vi "Move Addon Settings.vi"(8 "error in (no error)":errorcluster, 11 "Section Ref in":T1 format="%.0x") -> (0 "error out":errorcluster, 3 "Parent Ref out":T1 format="%.0x")   [LabVIEW 2023, in "J1939 Addon System Explorer.lvlib"]
uses:
  J1939 Addon System Explorer.lvlib
  <vilib>/NI VeriStand/Custom Device API/Custom Device Item Ref.ctl
  Addon Shared/SubVIs/Constants.vi
  <vilib>/NI VeriStand/Custom Device API/Custom Device API.lvlib
  Addon Shared/J1939 Addon Shared.lvlib
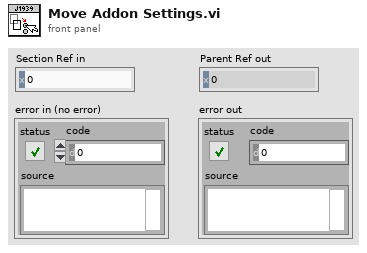
[diagram p1: front panel]
types:
  T1 = typedef "Custom Device API.lvlib/Custom Device Item Ref.ctl" = u64
  T2 = typedef "J1939 Addon Shared.lvlib/SPN Properties.ctl" = cluster{"Bytes":u32, "ScaleFac":dbl, "ScaleOff":dbl}
  T3 = cluster{"Name":string, "ID":u32, "Signal List":cluster{"Name":string, "SPN":T2}[]}[]
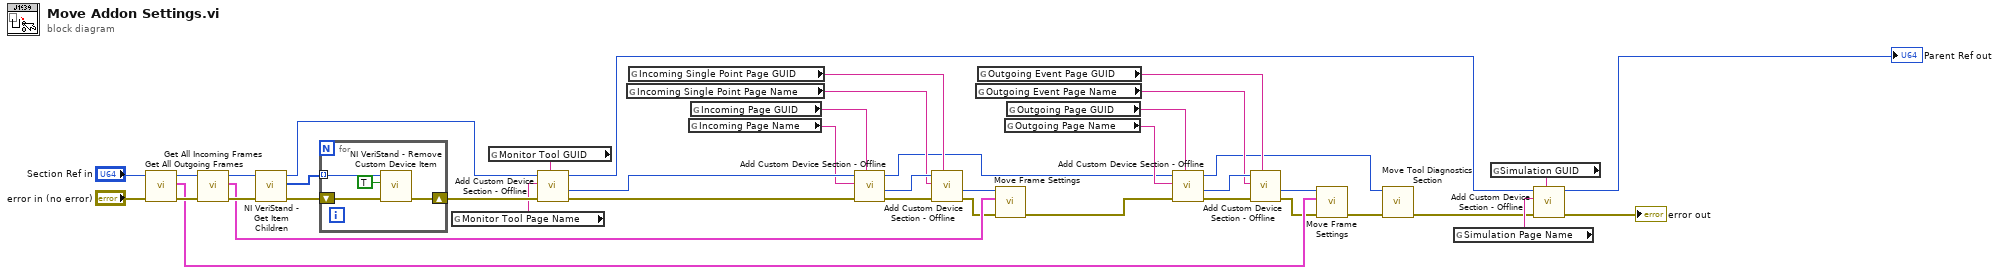
[diagram p0: block diagram]
diagram:
  n1 = call "Get All Outgoing Frames.vi"("error in"="error in (no error)", "Item Ref"="Section Ref in") -> ("error out"=w33:errorcluster, "Frames"=w29:T3, "Item Ref out"=w34:T1)  [unwired: 7 in]
  n2 = call "Get All Incoming Frames.vi"("error in"=w33, "Item Ref"=w34) -> ("error out"=w32:errorcluster, "Frames"=w30:T3, "Item Ref out"=w31:T1)  [unwired: 7 in]
  n3 = call <vilib>:"NI VeriStand - Get Item Children.vi"("error in (no error)"=w32, "Item Ref in"=w31) -> ("error out"=w38:errorcluster, "Child Refs"=w37:T1[], "Item Ref out"=w42:T1)  [unwired: 6 in, 1 out]
  n4 = for {
    tunnel: w37 -> [w46] mode=indexing
    shift-right: [w43] -> w41
    shift-left: w38 -> [w44]
    n5 = call <vilib>:"NI VeriStand - Remove Custom Device Item.vi"("error in (no error)"=w44, "Force Delete (F)"=TRUE, "Item Ref in"=w46) -> ("error out"=w43:errorcluster)  [unwired: 7 in, 1 out]
  }
  n6 = global read "Constants.vi" "Monitor Tool Page Name"() -> (w40:string)
  n7 = global read "Constants.vi" "Monitor Tool GUID"() -> (w39:string)
  n8 = call "Add Custom Device Section - Offline.vi"("GUID (Default Section)"=w39, "error in (no error)"=w41, "Section Name"=w40, "Parent Ref in"=w42) -> ("error out"=w28:errorcluster, "Section Ptr"=w27:T1, "Parent Ref out"=w2:T1)  [unwired: 4 in, 1 out]
  n9 = global read "Constants.vi" "Incoming Single Point Page Name"() -> (w21:string)
  n10 = global read "Constants.vi" "Incoming Single Point Page GUID"() -> (w22:string)
  n11 = global read "Constants.vi" "Incoming Page Name"() -> (w23:string)
  n12 = global read "Constants.vi" "Incoming Page GUID"() -> (w24:string)
  n13 = call "Add Custom Device Section - Offline.vi"("GUID (Default Section)"=w24, "error in (no error)"=w28, "Section Name"=w23, "Parent Ref in"=w27) -> ("error out"=w26:errorcluster, "Section Ptr"=w25:T1, "Parent Ref out"=w14:T1)  [unwired: 4 in, 1 out]
  n14 = call "Add Custom Device Section - Offline.vi"("GUID (Default Section)"=w22, "error in (no error)"=w26, "Section Name"=w21, "Parent Ref in"=w25) -> ("error out"=w10:errorcluster, "Section Ptr"=w12:T1)  [unwired: 4 in, 2 out]
  n15 = global read "Constants.vi" "Outgoing Event Page Name"() -> (w15:string)
  n16 = global read "Constants.vi" "Outgoing Event Page GUID"() -> (w16:string)
  n17 = call "Move Frame Settings.vi"("error in (no error)"=w10, "Frames"=w30, "Ref in"=w12) -> ("error out"=w9:errorcluster)  [unwired: 7 in, 1 out]
  n18 = global read "Constants.vi" "Outgoing Page Name"() -> (w17:string)
  n19 = global read "Constants.vi" "Outgoing Page GUID"() -> (w18:string)
  n20 = call "Add Custom Device Section - Offline.vi"("GUID (Default Section)"=w18, "error in (no error)"=w9, "Section Name"=w17, "Parent Ref in"=w14) -> ("error out"=w20:errorcluster, "Section Ptr"=w19:T1, "Parent Ref out"=w13:T1)  [unwired: 4 in, 1 out]
  n21 = call "Add Custom Device Section - Offline.vi"("GUID (Default Section)"=w16, "error in (no error)"=w20, "Section Name"=w15, "Parent Ref in"=w19) -> ("error out"=w8:errorcluster, "Section Ptr"=w11:T1)  [unwired: 4 in, 2 out]
  n22 = call "Move Frame Settings.vi"("error in (no error)"=w8, "Frames"=w29, "Ref in"=w11) -> ("error out"=w7:errorcluster)  [unwired: 7 in, 1 out]
  n23 = call "Move Tool Diagnostics Section.vi"("error in (no error)"=w7, "Device Item Ref in"=w13) -> ("error out"=w4:errorcluster)  [unwired: 8 in, 1 out]
  n24 = global read "Constants.vi" "Simulation Page Name"() -> (w6:string)
  n25 = global read "Constants.vi" "Simulation GUID"() -> (w5:string)
  n26 = call "Add Custom Device Section - Offline.vi"("GUID (Default Section)"=w5, "error in (no error)"=w4, "Section Name"=w6, "Parent Ref in"=w2) -> ("error out"=→"error out":errorcluster, "Parent Ref out"=→"Parent Ref out":T1)  [unwired: 4 in, 2 out]
